vi "GetDisplayTextState.vi"(8 "Error In":errorcluster, 10 "Window":u8=1 min=1 max=2 step=1, 11 "Keithley 6482 In":refnum<visa-resource-name>) -> (0 "Error Out":errorcluster, 2 "Enabled?":bool, 3 "Keithley 6482 Out":refnum<visa-resource-name>)   [LabVIEW 2012, in "Keithley-6482.lvlib"]
uses:
  Keithley-6482.lvlib
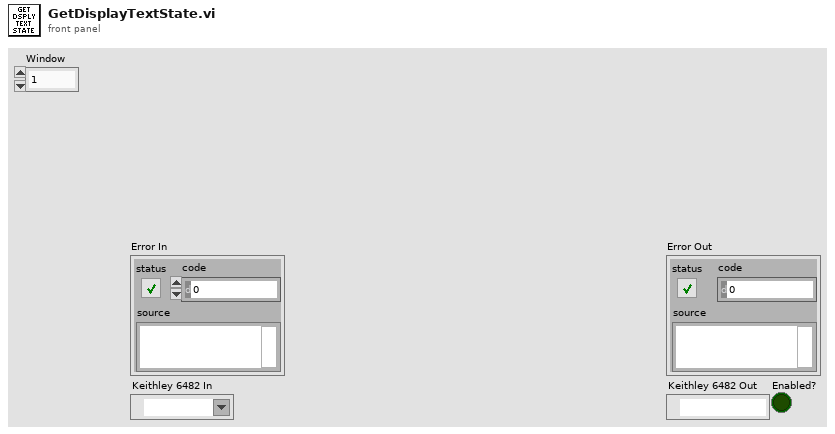
[diagram p1: front panel]
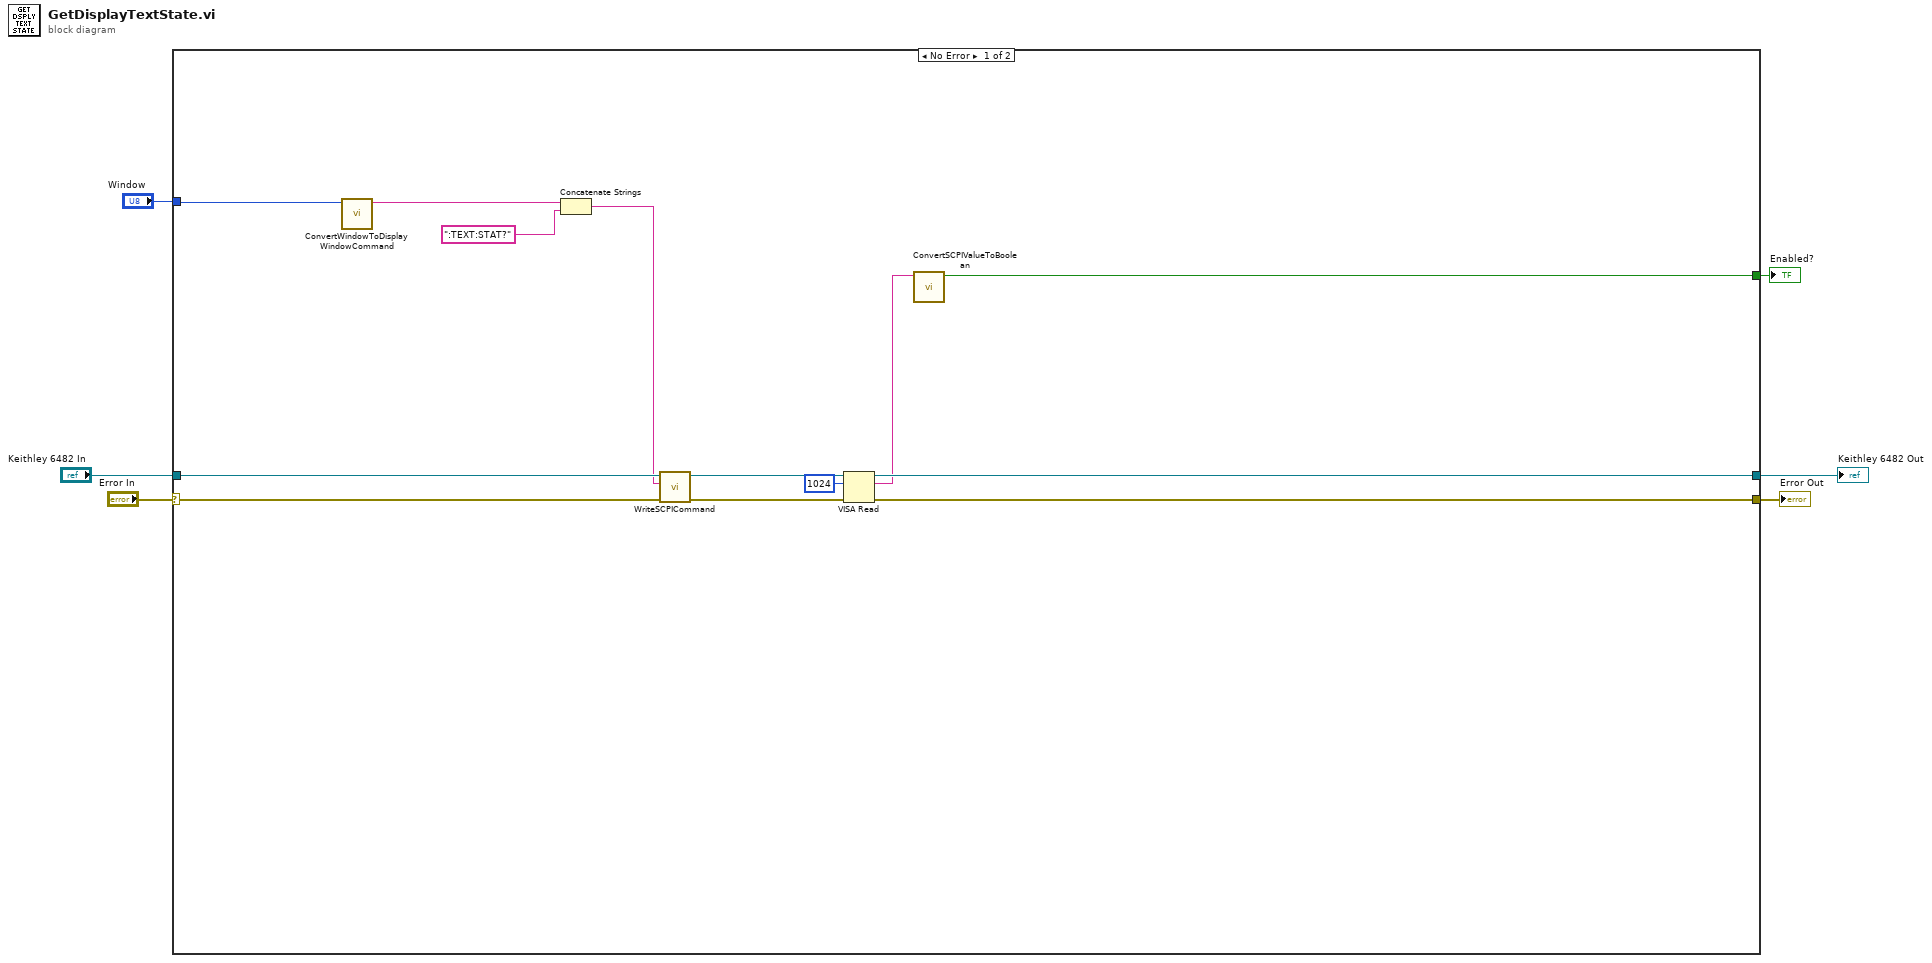
[diagram p0: block diagram]
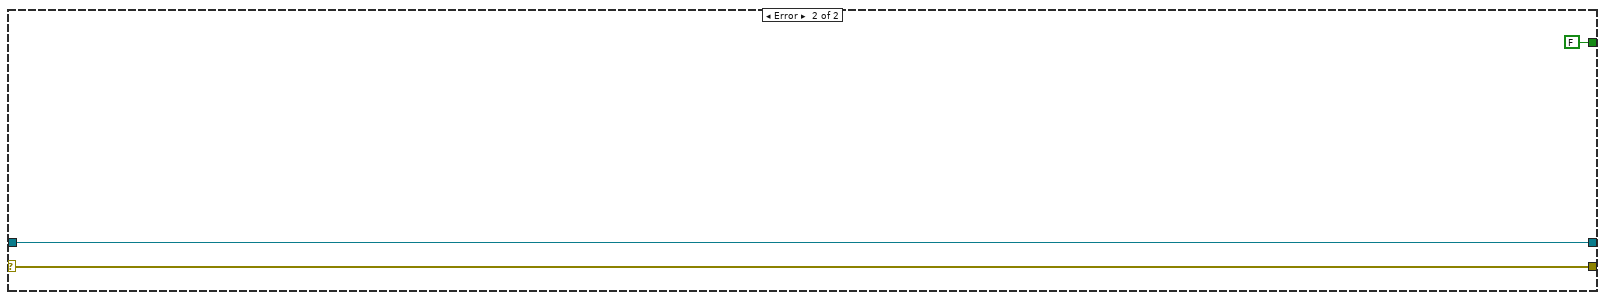
[diagram p2: hidden frame]
diagram:
  n1 = case shown="No Error" "Error In" {
    selector: "Error In" -> [w11 w21]
    tunnel: [w19 w21] -> w5
    tunnel: [w18 w22] -> w4
    tunnel: "Keithley 6482 In" -> [w12 w22]
    tunnel: [w15 FALSE ("Boolean")] -> w2
    tunnel: "Window" -> [w7 _]
    frame No Error {
      n2 = call "ConvertWindowToDisplayWindowCommand.vi"("Window"=w7) -> ("Display Window Command"=w8:string)  [unwired: 10 in]
      n3 = Concatenate Strings(w8, ":TEXT:STAT?") -> (w9:string)
      n4 = call "WriteSCPICommand.vi"("Error In"=w11, "SCPI Command"=w9, "Keithley 6482 In"=w12) -> ("Error Out"=w13:errorcluster, "Keithley 6482 Out"=w14:refnum<visa-resource-name>)  [unwired: 7 in]
      n5 = VISA Read(VISA resource name=w14, byte count=u32 1024, error in (no error)=w13) -> (VISA resource name out=w18:refnum<visa-resource-name>, read buffer=w16:string, error out=w19:errorcluster)  [unwired: 1 out]
      n6 = call "ConvertSCPIValueToBoolean.vi"("SCPI Value"=w16) -> ("Boolean"=w15:bool)  [unwired: 10 in]
    }
    frame Error {
    }
  }
  "Error Out" <- w5
  "Keithley 6482 Out" <- w4
  "Enabled?" <- w2
